vi "FTW-Benchmark-Actors.vi"() -> ()   [LabVIEW 2013]
uses:
  source/actor/Connector/FTW-ActorConnector.lvclass
panel:
  in  "Inbox Address":string(combo)="inproc://*"
  out "Actor Pool Spawn":dbl format="Actor Pool Spawn: %_3psec"
  out "Overall Pass?":bool
  out "Total Elapsed Time":dbl format="Messaging Time: %_3psec"
  out "\"FTW: Ping\" Times":cluster{dbl[]}[](graph)
  out "Results":T1(array[cluster])
  in  "Test to Perform":T2(radio)=enum."Parallel: 10x10"
  out "\"PING\" Times":cluster{dbl[]}[](graph)
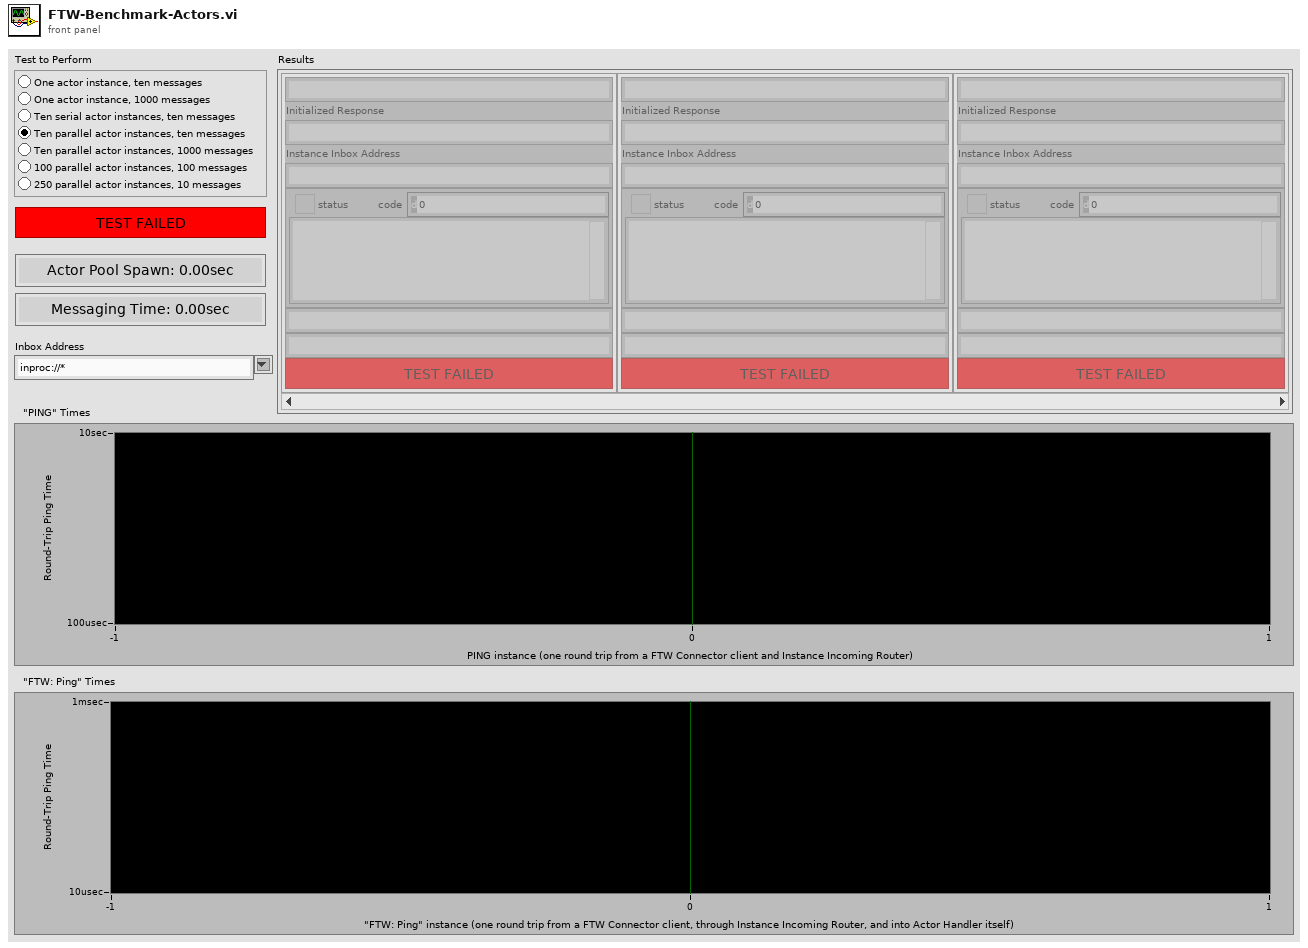
[diagram p1: front panel]
types:
  T1 = cluster{"Server Address":string, "Initialized Response":string, "Instance Inbox Address":string, "Error":errorcluster, "Server Address":string, "Server Address":string, "Pass?":bool}[]
  T2 = enum32{"Serial: 1x10", "Serial: 1x1000", "Serial: 10x10", "Parallel: 10x10", "Parallel: 10x100", "Parallel: 100x100", "Parallel: 250x10"}
  T3 = cluster{i32, "Initialized Response":string, "Instance Inbox Address":string, "error out":errorcluster}
  T4 = cluster{i32, bool, bool, "Timed out?":bool, cluster{dbl[]}, cluster{dbl[]}, "error out":errorcluster}
  T5 = cluster{string, "Initialized Response":string, "Instance Inbox Address":string, "error out":errorcluster, string, string, bool}
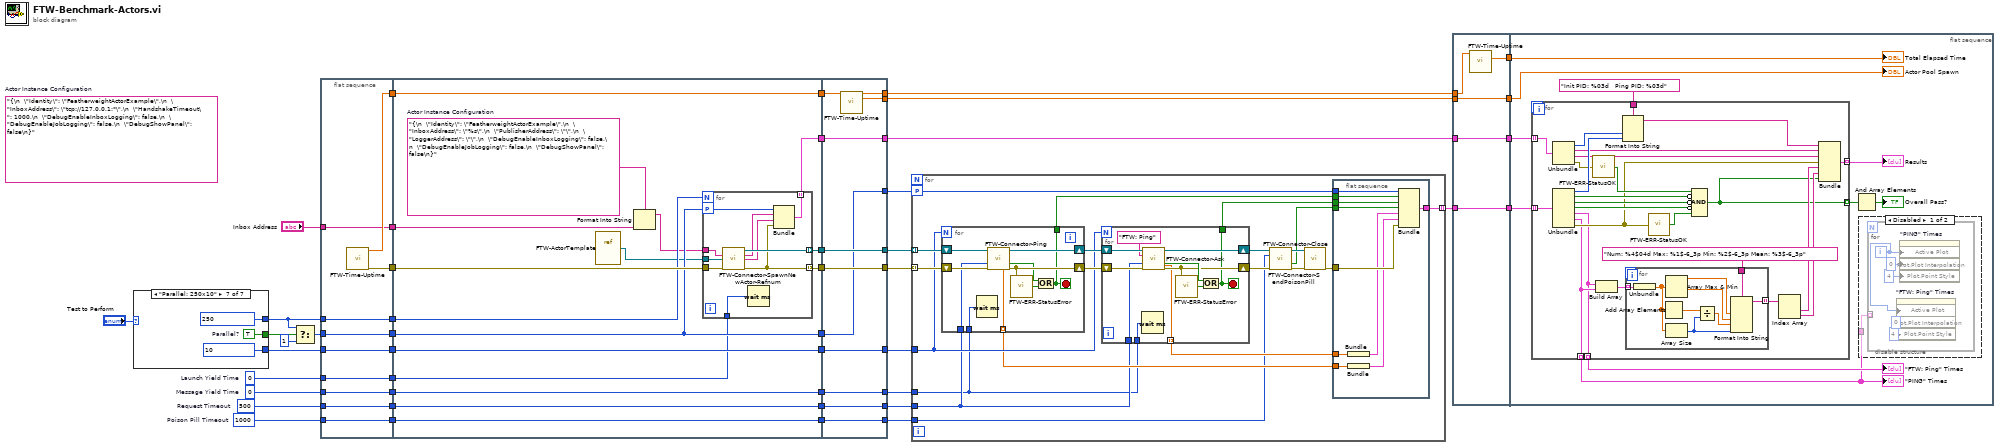
[diagram p0: block diagram]
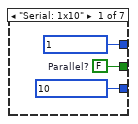
[diagram p2: hidden frame]
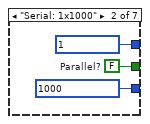
[diagram p3: hidden frame]
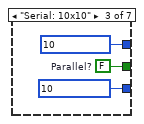
[diagram p4: hidden frame]
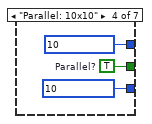
[diagram p5: hidden frame]
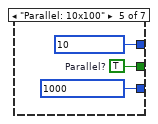
[diagram p6: hidden frame]
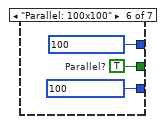
[diagram p7: hidden frame]
diagram:
  (unwired) "{\n  \"Identity\": \"FeatherweightActorExample\",\n  \"InboxAddress\": \"tcp://127.0.0.1:*\",\n  \"HandshakeTimeout\": 1000,\n  \"DebugEnableInboxLogging\": false,\n  \"DebugEnableJobLogging\": false,\n  \"DebugShowPanel\": false\n}"  # Actor Instance Configuration
  w3 = u32 0  # Message Yield Time
  w7 = u32 0  # Launch Yield Time
  w9 = 1000  # Poison Pill Timeout
  w11 = 500  # Request Timeout
  n1 = case shown="\"Parallel: 250x10\"" "Test to Perform" {
    tunnel: [1 1 10 10 10 100 250] -> w16
    tunnel: [10 1000 10 10 1000 100 10] -> w14
    tunnel: [w46 w49 w52 w55 w58 w61 w64] -> w20
    frame "Serial: 1x10" {
      w46 = FALSE  # Parallel?
    }
    frame "Serial: 1x1000" {
      w49 = FALSE  # Parallel?
    }
    frame "Serial: 10x10" {
      w52 = FALSE  # Parallel?
    }
    frame "Parallel: 10x10" {
      w55 = TRUE  # Parallel?
    }
    frame "Parallel: 10x100" {
      w58 = TRUE  # Parallel?
    }
    frame "Parallel: 100x100" {
      w61 = TRUE  # Parallel?
    }
    frame "Parallel: 250x10" {
      w64 = TRUE  # Parallel?
    }
  }
  n2 = Select(t=w16, s=w20, f=1) -> (s? t:f=w18:i32)
  n3 = flat-sequence {
    tunnel: [w76] -> w24
    tunnel: [w72] -> w23
    tunnel: [w75] -> w19
    tunnel: w18 -> [w75]
    tunnel: [w74] -> w17
    tunnel: w16 -> [w74]
    tunnel: [w73] -> w15
    tunnel: w14 -> [w73]
    tunnel: [w71] -> w12
    tunnel: w11 -> [w71]
    tunnel: [w70] -> w10
    tunnel: w9 -> [w70]
    tunnel: [w69] -> w8
    tunnel: w7 -> [w69]
    tunnel: [w68] -> w4
    tunnel: w3 -> [w68]
    tunnel: "Inbox Address" -> [w67]
    tunnel: [w67] -> w1
    tunnel: [w92] -> w36
    tunnel: [w91] -> w35
    tunnel: [w85] -> w34
    tunnel: [w87] -> w33
    tunnel: [w90] -> w32
    tunnel: [w88] -> w31
    tunnel: [w84] -> w27
    tunnel: [w83] -> w25
    tunnel: w24 -> [w89]
    tunnel: w23 -> [w88]
    tunnel: w19 -> [w87]
    tunnel: w17 -> [w86]
    tunnel: w15 -> [w85]
    tunnel: w12 -> [w84]
    tunnel: w10 -> [w83]
    tunnel: w8 -> [w82]
    tunnel: [w81] -> w5
    tunnel: w4 -> [w81]
    tunnel: w1 -> [w78]
    tunnel: [w109] -> w41
    tunnel: [w110] -> w42
    tunnel: [w111] -> w43
    tunnel: [w112] -> w44
    tunnel: [w113] -> w45
    tunnel: w36 -> [w113]
    tunnel: w35 -> [w112]
    tunnel: w34 -> [w111]
    tunnel: w33 -> [w110]
    tunnel: w32 -> [w109]
    tunnel: w31 -> [w108]
    tunnel: [w107] -> w29
    tunnel: [w106] -> w28
    tunnel: w27 -> [w106]
    tunnel: [w105] -> w26
    tunnel: w25 -> [w105]
    tunnel: [w104] -> w13
    tunnel: [w103] -> w6
    tunnel: w5 -> [w103]
    frame #0 {
      n4 = call "FTW-Time-Uptime.vi"() -> ("Current Uptime"=w72:dbl, "error out"=w76:errorcluster)  [unwired: 13 in, 1 out]
    }
    frame #1 {
      w80 = "{\n  \"Identity\": \"FeatherweightActorExample\",\n  \"InboxAddress\": \"%s\",\n  \"PublisherAddress\": \"\",\n  \"LoggerAddress\": \"\",\n  \"DebugEnableInboxLogging\": false,\n  \"DebugEnableJobLogging\": false,\n  \"DebugShowPanel\": false\n}"  # Actor Instance Configuration
      n5 = vi-ref "FTW-ActorTemplate.vi"() -> (w77:refnum<vi>)
      n6 = Format Into String(format string=w80, w78) -> (resulting string=w79:string)  [unwired: 2 in, 1 out]
      n7 = for {
        N: w86 -> [_]
        tunnel: w79 -> [w95]
        tunnel: w89 -> [w102]
        tunnel: [w101] -> w92 mode=indexing
        tunnel: [w97] -> w91 mode=indexing
        tunnel: [w98] -> w90 mode=indexing
        workers-P: w87 -> [w96]
        tunnel: w82 -> [w94]
        tunnel: w77 -> [w93]
        n8 = call "FTW-Connector-SpawnNewActor-Refnum.vi"("Configuration"=w95, "Actor VI Refnum"=w93, "error in"=w102) -> ("FTW Actor Connector"=w101:refnum<class "FTW-ActorConnector.lvclass">, "Initialized Response"=w100:string, "Instance Inbox Address"=w99:string, "error out"=w97:errorcluster)  [unwired: 9 in]
        n9 = Wait (ms)(milliseconds to wait=w94) -> ()  [unwired: 1 out]
        n10 = Bundle(w96, "Initialized Response"=w100, "Instance Inbox Address"=w99, "error out"=w97) -> (w98:T3)  [unwired: 1 in]
      }
    }
    frame #2 {
      n11 = call "FTW-Time-Uptime.vi"("Previous Uptime"=w108) -> ("Current Uptime"=w104:dbl, "Elapsed Time"=w107:dbl)  [unwired: 12 in, 1 out]
    }
  }
  n12 = for {
    tunnel: w45 -> [w131] mode=indexing
    tunnel: w44 -> [w130] mode=indexing
    tunnel: w43 -> [w125]
    workers-P: w42 -> [w124]
    tunnel: [w121] -> w40 mode=indexing
    tunnel: w28 -> [w117]
    tunnel: w26 -> [w116]
    tunnel: w6 -> [w115]
    n13 = for {
      N: w125 -> [_]
      tunnel: [w151] -> w118 mode=indexing
      shift-right: [w152] -> w129
      shift-left: w131 -> [w154]
      shift-right: [w150] -> w128
      shift-left: w130 -> [w153]
      tunnel: [w147] -> w123
      tunnel: w117 -> [w146]
      tunnel: w115 -> [w145]
      stop <- w147 stop-if-true
      n14 = Wait (ms)(milliseconds to wait=w145) -> ()  [unwired: 1 out]
      n15 = call "FTW-Connector-Ping.vi"("FTW Actor Connector"=w154, "Timeout"=w146, "error in"=w153) -> ("FTW Actor Connector out"=w152:refnum<class "FTW-ActorConnector.lvclass">, "Timed out?"=w148:bool, "Roundtrip Time"=w151:dbl, "error out"=w150:errorcluster)  [unwired: 8 in, 1 out]
      n16 = call "FTW-ERR-StatusError.vi"("error to check"=w150) -> ("Error?"=w149:bool)
      n17 = Or(x=w148, y=w149) -> (x .or. y?=w147:bool)
    }
    n18 = for {
      N: w125 -> [_]
      tunnel: [w139] -> w119 mode=indexing
      shift-right: [w142] -> w127
      shift-left: w129 -> [w143]
      shift-right: [w140] -> w126
      shift-left: w128 -> [w138]
      tunnel: [w137] -> w122
      tunnel: w117 -> [w136]
      tunnel: w115 -> [w135]
      stop <- w137 stop-if-true
      n19 = Wait (ms)(milliseconds to wait=w135) -> ()  [unwired: 1 out]
      n20 = call "FTW-Connector-Ask.vi"("FTW Actor Connector"=w143, "Request Header"="FTW: Ping", "Timeout"=w136, "error in"=w138) -> ("FTW Actor Connector out"=w142:refnum<class "FTW-ActorConnector.lvclass">, "Timed out?"=w141:bool, "Roundtrip Time"=w139:dbl, "error out"=w140:errorcluster)  [unwired: 5 in, 3 out]
      n21 = call "FTW-ERR-StatusError.vi"("error to check"=w140) -> ("Error?"=w144:bool)
      n22 = Or(x=w141, y=w144) -> (x .or. y?=w137:bool)
    }
    n23 = call-dynamic "FTW-Connector-SendPoisonPill.vi"("FTW Actor Connector"=w127, "Timeout"=w116, "error in"=w126) -> ("FTW Actor Connector out"=w133:refnum<class "FTW-ActorConnector.lvclass">, "Timed out?"=w114:bool, "error out"=w132:errorcluster)  [unwired: 8 in, 2 out]
    n24 = call-dynamic "FTW-Connector-Close.vi"("FTW Actor Connector"=w133, "error in"=w132) -> ("error out"=w120:errorcluster)  [unwired: 13 in]
    n25 = flat-sequence {
      tunnel: w124 -> [w164]
      tunnel: w123 -> [w163]
      tunnel: w122 -> [w162]
      tunnel: [w161] -> w121
      tunnel: w114 -> [w160]
      tunnel: w120 -> [w159]
      tunnel: w119 -> [w157]
      tunnel: w118 -> [w155]
      frame #0 {
        n26 = Bundle(w157) -> (w158:cluster{dbl[]})  [unwired: 1 in]
        n27 = Bundle(w155) -> (w156:cluster{dbl[]})  [unwired: 1 in]
        n28 = Bundle(w164, w163, w162, "Timed out?"=w160, w158, w156, "error out"=w159) -> (w161:T4)  [unwired: 1 in]
      }
    }
  }
  n29 = flat-sequence {
    tunnel: w40 -> [w168]
    tunnel: w41 -> [w169]
    tunnel: [w169] -> w39
    tunnel: [w168] -> w38
    tunnel: [w167] -> w37
    tunnel: [w166] -> w30
    tunnel: w29 -> [w166]
    tunnel: w13 -> [w165]
    tunnel: w39 -> [w179]
    tunnel: w38 -> [w178]
    tunnel: w37 -> [w174]
    tunnel: w30 -> [w171]
    frame #0 {
      n30 = call "FTW-Time-Uptime.vi"("Previous Uptime"=w165) -> ("Elapsed Time"=w167:dbl)  [unwired: 12 in, 2 out]
    }
    frame #1 {
      n31 = for {
        tunnel: w179 -> [w209] mode=indexing
        tunnel: w178 -> [w208] mode=indexing
        tunnel: "Init PID: %03d   Ping PID: %03d" ("format string") -> [w207]
        tunnel: [w191] -> w176 mode=indexing
        tunnel: [w187] -> w175 mode=indexing
        tunnel: [w190] -> w170 mode=indexing
        tunnel: [w189] -> w173 mode=indexing
        n32 = Unbundle(w209) -> (w206:i32, "Initialized Response"=w198:string, "Instance Inbox Address"=w197:string, "error out"=w186:errorcluster)
        n33 = Unbundle(w208) -> (w205:i32, w203:bool, w202:bool, "Timed out?"=w201:bool, w187:cluster{dbl[]}, w190:cluster{dbl[]}, "error out"=w196:errorcluster)
        n34 = call "FTW-ERR-StatusOK.vi"("error to check"=w186) -> ("Status OK?"=w204:bool)
        n35 = Build Array(w187, w190) -> (w195:cluster{dbl[]}[])
        n36 = Format Into String(format string=w207, w206, w205) -> (resulting string=w199:string)  [unwired: 2 in, 1 out]
        n37 = for {
          tunnel: w195 -> [w214] mode=indexing
          tunnel: [w212] -> w194 mode=indexing
          tunnel: "Num: %4$04d Max: %1$-6_3p Min: %2$-6_3p Mean: %3$-6_3p" ("format string") -> [w211]
          n38 = Unbundle(w214) -> (w213:dbl[])
          n39 = Add Array Elements(numeric array=w213) -> (sum=w218:dbl)
          n40 = Array Max & Min(array=w213) -> (max value=w217:dbl, min value=w216:dbl)  [unwired: 2 out]
          n41 = Array Size(array=w213) -> (size(s)=w210:i32)
          n42 = Divide(x=w218, y=w210) -> (x/y=w215:dbl)
          n43 = Format Into String(format string=w211, w217, w216, w215, w210) -> (resulting string=w212:string)  [unwired: 2 in, 1 out]
        }
        n44 = call "FTW-ERR-StatusOK.vi"("error to check"=w196) -> ("Status OK?"=w200:bool)
        n45 = Compound Arithmetic op=AND(w204, invert w203, invert w202, invert w201, w200) -> (w189:bool)
        n46 = Index Array(array=w194) -> (element #1=w193:string, element #2=w192:string)  [unwired: 2 in]
        n47 = Bundle(w199, "Initialized Response"=w198, "Instance Inbox Address"=w197, "error out"=w196, w193, w192, w189) -> (w191:T5)  [unwired: 1 in]
      }
      "\"PING\" Times" <- w170
      "Results" <- w176
      "\"FTW: Ping\" Times" <- w175
      n48 = And Array Elements(Boolean array=w173) -> (logical AND=→"Overall Pass?":bool)
      n49 = disable-structure shown="Disabled" {
        disable-tunnel: w170 -> [w180 _]
        frame Disabled {
          n50 = for {
            tunnel: w180 -> [_] mode=indexing
            i -> [w181]
            n51 = property on="\"FTW: Ping\" Times" class="WFGraph (strict)"("Active Plot"=w181, "Plot.Plot Interpolation"=u8 0 ("Plot.Line Style"), "Plot.Point Style"=u8 4) -> ()  [unwired: 2 in, 2 out]
            n52 = property on="\"PING\" Times" class="WFGraph (strict)"("Active Plot"=w181, "Plot.Plot Interpolation"=u8 0 ("Plot.Line Style"), "Plot.Point Style"=u8 4) -> ()  [unwired: 2 in, 2 out]
          }
        }
        frame Enabled {
        }
      }
      "Total Elapsed Time" <- w174
      "Actor Pool Spawn" <- w171
    }
  }
